vi "SAG_delay_flag_G4.vi"(11 "ID_EQUIPO":i32) -> ()   [LabVIEW 2018]
uses:
  Global/PQ_flags.vi
panel:
  out "time sag":dbl
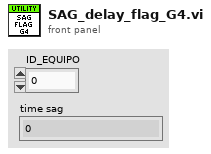
[diagram p1: front panel]
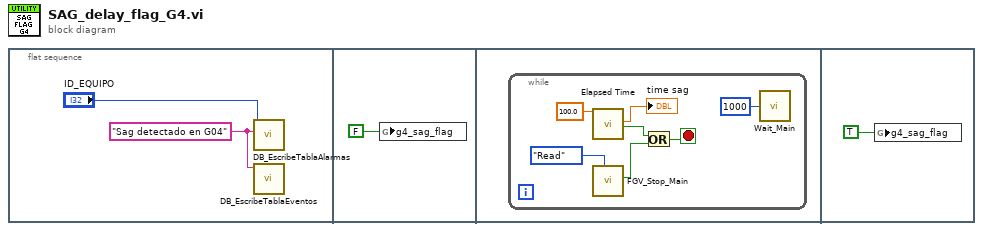
[diagram p0: block diagram]
diagram:
  n1 = flat-sequence {
    frame #0 {
      w1 = "Sag detectado en G04" ("MOTIVO")
      n2 = call "DB_EscribeTablaAlarmas.vi"("MOTIVO"=w1, "ID_EQUIPO"="ID_EQUIPO") -> ()  [unwired: 9 in, 1 out]
      n3 = call "DB_EscribeTablaEventos.vi"("DESCRIPCION"=w1) -> ()  [unwired: 10 in, 1 out]
    }
    frame #1 {
      n4 = global write "PQ_flags.vi" "g4_sag_flag"(FALSE ("sag_flag")) -> ()
    }
    frame #2 {
      n5 = while {
        stop <- w7 stop-if-true
        n6 = call "Elapsed Time"("Time Target (s)"=100.0) -> ("Elapsed Time (s)"=→"time sag":dbl, "Time has Elapsed"=w6:bool)  [unwired: 11 in, 6 out]
        n7 = call "FGV_Stop_Main.vi"("Action"=enum16{"Read", "Write"}."Read") -> ("Var Out"=w4:bool)  [unwired: 9 in, 1 out]
        n8 = Or(x=w6, y=w4) -> (x .or. y?=w7:bool)
        n9 = call "Wait_Main.vi"("Wait time (msec)"=u32 1000) -> ()  [unwired: 5 in]
      }
    }
    frame #3 {
      n10 = global write "PQ_flags.vi" "g4_sag_flag"(TRUE ("sag_flag")) -> ()
    }
  }
